vi "VI_unlock.vi"(6 "Verify salt (T)":bool=TRUE, 7 "Remove lib password (T)":bool=TRUE, 8 "error in (no error)":errorcluster, 9 "New Password (\"\")":string, 10 "Output file":path, 11 "Input file":path) -> (0 "error out":errorcluster, 1 "Hash1 salt":string, 2 "Icon":picture, 3 "Version string":string, 4 "Bruteforced salt":bool)   [LabVIEW 2020]
uses:
  <vilib>/Utility/error.llb/Trim Whitespace One-Sided.vi
panel:
  # "(Disable to repair broken BDPW hashes)"
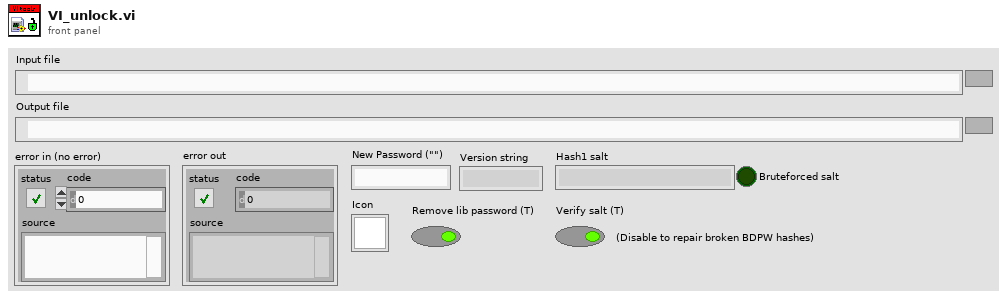
[diagram p1: front panel]
types:
  T1 = cluster{"Major":u8, "Minor":u8, "Fix":u8, "Build":u8}
  T2 = enum16{"open", "replace", "create", "open or create", "replace or create", "replace or create with confirmation"}
  T3 = map{string, cluster{"Offset":i32, "Data":string}}
  T4 = cluster{"Hash1 raw (no salt)":string, "Hash1 (MD5)":string}
  T5 = cluster{"version":u32, "Flags":u32, "viFlags2":u32, "viFlags0C":u32, "viFlags10":u32, "buttonsHidden":u16, "frontpFlags":u16, "instrState":u32, "execState":u32, "execPrio":u16, "viType":u16, "prefExecSyst":i32, "field28":u32, "field2C":u32, "field30":u32, "viSignatureHi":u64, "viSignatureLo":u64, "alignGridFP":u32, "alignGridBD":u32, "field4C":u16, "ctrlIndStyle":u16, "field50_md5Hi":u64, "field50_md5Lo":u64, "libHi":u64, "libLo":u64}
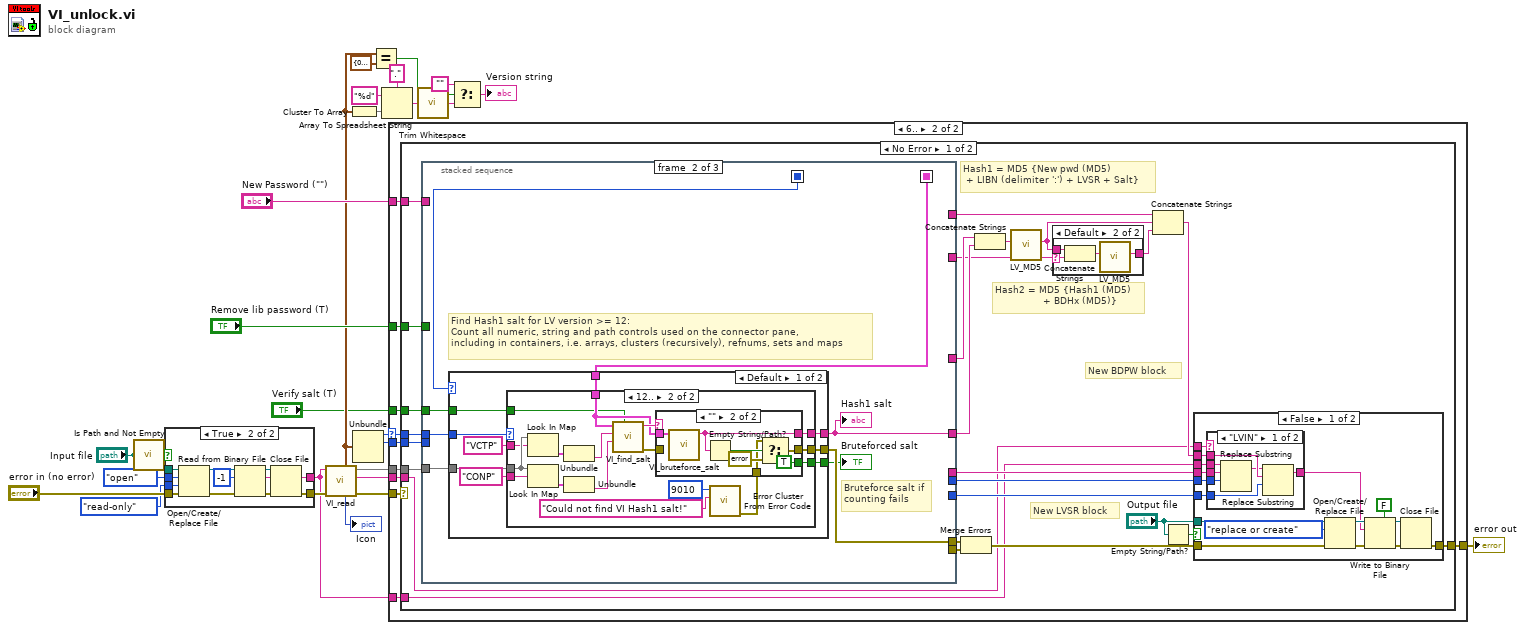
[diagram p0: block diagram]
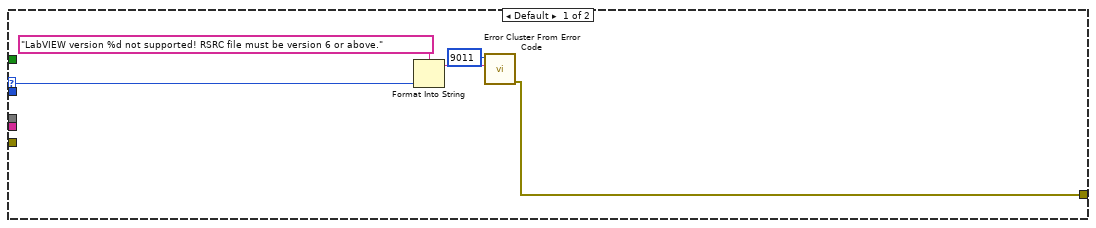
[diagram p2: hidden frame]
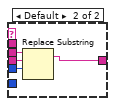
[diagram p4: hidden frame]
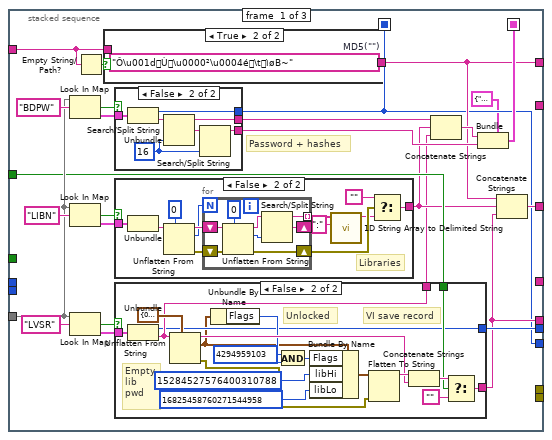
[diagram p6: hidden frame]
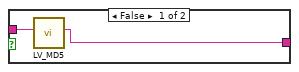
[diagram p7: hidden frame]
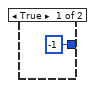
[diagram p8: hidden frame]
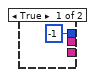
[diagram p10: hidden frame]
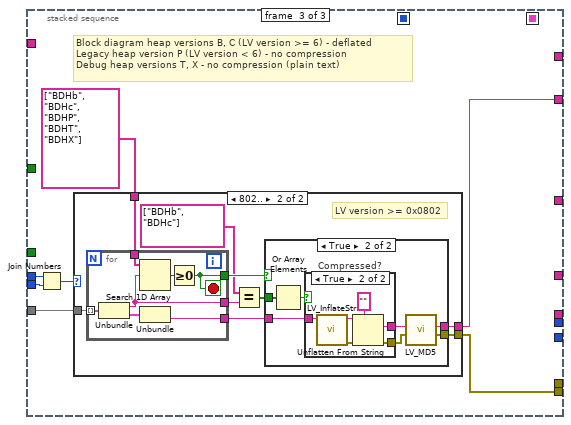
[diagram p14: hidden frame]
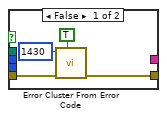
[diagram p19: hidden frame]
diagram:
  n1 = call <vilib>:"Is Path and Not Empty.vi"("path"="Input file") -> ("Is Path and Not Empty?"=w19:bool)  [unwired: 4 in]
  n2 = case "Empty?" shown="True" w19 {
    tunnel: "error in (no error)" -> [w31 w42]
    tunnel: "Input file" -> [_ w41]
    tunnel: [w28 w32] -> w27
    tunnel: enum16{"read/write", "read-only", "write-only"}."read-only" ("access (0:read/write)") -> [_ w40]
    tunnel: T2."open" ("operation (0:open)") -> [_ w39]
    tunnel: [_ w35] -> w5
    frame False {
      n3 = call <vilib>:"Error Cluster From Error Code.vi"("show call chain? (False)"=TRUE, "error in (no error)"=w31, "error code (0)"=1430) -> ("error out"=w28:errorcluster)  [unwired: 6 in]
    }
    frame True {
      n4 = Open/Create/Replace File(file path (use dialog)=w41, error in=w42, operation (0:open)=w39, access (0:read/write)=w40) -> (refnum out=w37:refnum<file>, error out=w38:errorcluster)  [unwired: 2 in, 1 out]
      n5 = Read from Binary File(8:w38, 10:-1 ("count (1)"), 11:w37) -> (0:w33:errorcluster, 2:w35:string, 3:w34:refnum<file>)  [unwired: 3 in, 1 out]
      n6 = Close File(refnum=w34, error in=w33) -> (error out=w32:errorcluster)  [unwired: 1 out]
    }
  }
  n7 = call "VI_read.vi"("error in (no error)"=w27, "File bytestream"=w5) -> ("error out"=w23:errorcluster, "Resource type"=w18:string, "Blocks"=w21:T3, "Icon"=→"Icon":picture, "Version"=w4:T1)  [unwired: 5 in]
  n8 = Cluster To Array(cluster=w4) -> (array=w12:u8[])
  n9 = Unbundle(w4) -> ("Major"=w3:u8, "Minor"=w2:u8)  [unwired: 2 out]
  n10 = Equal?(x=w4, y=T1 {"Major"=0, "Minor"=0, "Fix"=0, "Build"=0}) -> (x = y?=w10:bool)
  n11 = Array To Spreadsheet String(delimiter (Tab)=".", array=w12, 3:"%d" ("format string")) -> (spreadsheet string=w13:string)
  n12 = case shown="6.." w3 {
    selector: w3 -> [w45 w50]
    tunnel: w23 -> [_ w57]
    tunnel: [w43 w56] -> w22
    tunnel: w21 -> [_ w55]
    tunnel: w18 -> [_ w54]
    tunnel: "New Password (\"\")" -> [_ w53]
    tunnel: "Remove lib password (T)" -> [_ w52]
    tunnel: w5 -> [_ w51]
    tunnel: w2 -> [_ w49]
    tunnel: "Verify salt (T)" -> [_ w48]
    frame Default {
      n13 = Format Into String(format string="LabVIEW version %d not supported! RSRC file must be version 6 or above.", w45) -> (resulting string=w44:string)  [unwired: 2 in, 1 out]
      n14 = call <vilib>:"Error Cluster From Error Code.vi"("error message (\"\")"=w44, "error code (0)"=9011) -> ("error out"=w43:errorcluster)  [unwired: 7 in]
    }
    frame 6.. {
      n15 = case shown="No Error" w57 {
        selector: w57 -> [_ w269]
        tunnel: w55 -> [w71 _]
        tunnel: w54 -> [w61 _]
        tunnel: [w62 w269] -> w56
        tunnel: w50 -> [w66 _]
        tunnel: w53 -> [w70 _]
        tunnel: w52 -> [w69 _]
        tunnel: w51 -> [w60 _]
        tunnel: w49 -> [w59 _]
        tunnel: w48 -> [w58 _]
        frame No Error {
          # "New BDPW block"
          # "New LVSR block"
          # "Hash2 = MD5 {Hash1 (MD5)\n                + BDHx (MD5)}"
          # "Hash1 = MD5 {New pwd (MD5)\n + LIBN (delimiter ':') + LVSR + Salt}"
          n16 = stacked-sequence {
            seq-local: [w121 _ _] -> [_ w194 _]
            seq-local: [w116 _ _] -> [_ w190 _]
            tunnel: [_ w192 _] -> w76
            tunnel: w70 -> [w124 _ _]
            tunnel: [_ _ w238] -> w65
            tunnel: [w126 _ _] -> w78
            tunnel: [w119 _ _] -> w77
            tunnel: [w116 _ _] -> w64
            tunnel: [_ _ w237] -> w81
            tunnel: w71 -> [w131 w193 w236]
            tunnel: w69 -> [w127 _ _]
            tunnel: [w118 _ _] -> w68
            tunnel: [w117 _ _] -> w67
            tunnel: w66 -> [_ w196 w234]
            tunnel: [_ w195 _] -> w82
            tunnel: w59 -> [_ _ w233]
            tunnel: w58 -> [_ w189 _]
            frame #0 {
              # "Password + hashes"
              n17 = Look In Map(map=w131, key="BDPW") -> (key not found?=w137:bool, value=w136:cluster{"Offset":i32, "Data":string})  [unwired: 1 in]
              n18 = Look In Map(map=w131, key="LIBN") -> (key not found?=w134:bool, value=w133:cluster{"Offset":i32, "Data":string})  [unwired: 1 in]
              n19 = Look In Map(map=w131, key="LVSR") -> (key not found?=w129:bool, value=w128:cluster{"Offset":i32, "Data":string})  [unwired: 1 in]
              n20 = Empty String/Path?(string/path=w124) -> (empty?=w125:bool)
              n21 = case shown="True" w125 {
                tunnel: w124 -> [w140 _]
                tunnel: [w139 w141] -> w118
                frame False {
                  n22 = call "LV_MD5.vi"("Input string"=w140) -> ("MD5 digest (16-bytes)"=w139:string)  [unwired: 9 in, 1 out]
                }
                frame True {
                  w141 = "Ô\u001dÙ\u0000²\u0004é\tìøB~"  # MD5("")
                }
              }
              n23 = case "Has BDPW?" shown="False" w137 {
                tunnel: w136 -> [_ w188]
                tunnel: [-1 ("Offset") w187] -> w116
                tunnel: [_ w183] -> w130
                tunnel: [_ w182] -> w122
                frame True {
                }
                frame False {
                  w184 = 16 ("offset (0)")
                  n24 = Unbundle(w188) -> ("Offset"=w187:i32, "Data"=w186:string)
                  n25 = Search/Split String(string=w186, offset (0)=w184) -> (substring before match=w183:string, match + rest of string=w185:string)  [unwired: 1 in, 1 out]
                  n26 = Search/Split String(string=w185, offset (0)=w184) -> (substring before match=w182:string)  [unwired: 1 in, 2 out]
                }
              }
              n27 = case "Has LIBN?" shown="False" w134 {
                tunnel: w133 -> [_ w168]
                tunnel: [_ w161] -> w120
                frame True {
                }
                frame False {
                  # "Libraries"
                  n28 = Unbundle(w168) -> ("Data"=w167:string)  [unwired: 1 out]
                  n29 = Unflatten From String(type=0 ("I32"), binary string=w167) -> (rest of the binary string=w170:string, value=w169:i32, error out=w171:errorcluster)  [unwired: 3 in]
                  n30 = for {
                    N: w169 -> [_]
                    shift-right: [w174] -> _
                    shift-left: w170 -> [w178]
                    shift-right: [w175] -> w164
                    shift-left: w171 -> [w179]
                    tunnel: [w173] -> w166 mode=indexing
                    n31 = Unflatten From String(type=u8 0 ("U8"), binary string=w178, error in (no error)=w179) -> (rest of the binary string=w177:string, value=w176:u8, error out=w175:errorcluster)  [unwired: 2 in]
                    n32 = Search/Split String(string=w177, offset (0)=w176) -> (substring before match=w173:string, match + rest of string=w174:string)  [unwired: 1 in, 1 out]
                  }
                  n33 = call <vilib>:"1D String Array to Delimited String.vi"("delimiter"=":", "string array"=w166) -> ("delimited string"=w163:string)  [unwired: 9 in]
                  n34 = Select(t="", s=w164, f=w163) -> (s? t:f=w161:string)
                }
              }
              n35 = case "Has LIBN?" shown="False" w129 {
                tunnel: w128 -> [_ w150]
                tunnel: [_ w146] -> w117
                tunnel: w127 -> [_ w148]
                tunnel: [-1 ("Offset") w144] -> w126
                tunnel: [_ w149] -> w115
                frame True {
                }
                frame False {
                  # "VI save record"
                  # "Unlocked"
                  # "Empty\nlib\npwd"
                  n36 = Unbundle(w150) -> ("Offset"=w144:i32, "Data"=w149:string)
                  n37 = Unflatten From String(type=T5 {"version"=0, "Flags"=0, "viFlags2"=0, "viFlags0C"=0, "viFlags10"=0, "buttonsHidden"=0, "frontpFlags"=0, "instrState"=0, "execState"=0, "execPrio"=0, "viType"=0, "prefExecSyst"=0, "field28"=0, "field2C"=0, "field30"=0, "viSignatureHi"=0, "viSignatureLo"=0, "alignGridFP"=0, "alignGridBD"=0, "field4C"=0, "ctrlIndStyle"=0, "field50_md5Hi"=0, "field50_md5Lo"=0, "libHi"=0, "libLo"=0} ("LVSR"), binary string=w149) -> (rest of the binary string=w157:string, value=w143:T5, error out=w145:errorcluster)  [unwired: 3 in]
                  n38 = Unbundle By Name(w143) -> ("Flags"=w147:u32)
                  n39 = And(x=u32 4294959103 ("Unlocked"), y=w147) -> (x .and. y?=w151:u32)
                  n40 = Bundle By Name(cluster=w143, "Flags"=w151, "libHi"=u64 15284527576400310788 ("libpass_md5Hi"), "libLo"=u64 16825458760271544958 ("libpass_md5Lo")) -> (w156:T5)
                  n41 = Flatten To String(anything=w156, error in (no error)=w145) -> (data string=w158:string)  [unwired: 2 in, 2 out]
                  n42 = Concatenate Strings(w158, w157) -> (w160:string)
                  n43 = Select(t=w160, s=w148, f="") -> (s? t:f=w146:string)
                }
              }
              n44 = Concatenate Strings(w130, w120, w115) -> (w123:string)
              n45 = Bundle(cluster=T4 {"Hash1 raw (no salt)"="", "Hash1 (MD5)"=""} ("output cluster"), "Hash1 raw (no salt)"=w123, "Hash1 (MD5)"=w122) -> (w121:T4)
              n46 = Concatenate Strings(w118, w120, w117) -> (w119:string)
            }
            frame #1 {
              # "Bruteforce salt if\ncounting fails"
              # "Find Hash1 salt for LV version >= 12:\nCount all numeric, string and path controls used on the connector pane,\nincluding in containers, i.e. arrays, clusters (recursively), refnums, sets and maps"
              n47 = case shown="Default" w190 {
                tunnel: [w205 _] -> w192
                tunnel: w196 -> [w202 _]
                tunnel: [w204 _] -> w195
                tunnel: w194 -> [w203 _]
                tunnel: w193 -> [w201 _]
                tunnel: [w199 _] -> w191
                tunnel: w189 -> [w197 _]
                frame Default {
                  n48 = case shown="12.." w202 {
                    tunnel: [_ w217] -> w205
                    tunnel: w203 -> [_ w207]
                    tunnel: [_ w218] -> w204
                    tunnel: w201 -> [_ w212]
                    tunnel: "CONP" ("key") -> [_ w221]
                    tunnel: [_ w213] -> w199
                    tunnel: "VCTP" ("key") -> [_ w211]
                    tunnel: w197 -> [_ w206]
                    frame Default {
                    }
                    frame 12.. {
                      n49 = Look In Map(map=w212, key=w211) -> (value=w210:cluster{"Offset":i32, "Data":string})  [unwired: 1 in, 1 out]
                      n50 = Look In Map(map=w212, key=w221) -> (value=w222:cluster{"Offset":i32, "Data":string})  [unwired: 1 in, 1 out]
                      n51 = Unbundle(w210) -> ("Data"=w209:string)  [unwired: 1 out]
                      n52 = Unbundle(w222) -> ("Data"=w208:string)  [unwired: 1 out]
                      n53 = call "VI_find_salt.vi"("Verify salt (T)"=w206, "CONP block"=w208, "VCTP block"=w209, "Hashes"=w207) -> ("error out"=w219:errorcluster, "Salt"=w220:string)  [unwired: 6 in]
                      n54 = call <vilib>:"Error Cluster From Error Code.vi"("error message (\"\")"="Could not find VI Hash1 salt!" ("error message (\"\")"), "error code (0)"=9010) -> ("error out"=w214:errorcluster)  [unwired: 7 in]
                      n55 = case shown="\"\"" w220 {
                        selector: w220 -> [w223 _]
                        tunnel: [w224 w226] -> w218
                        tunnel: w219 -> [w224 _]
                        tunnel: [w223 w230] -> w217
                        tunnel: w207 -> [_ w231]
                        tunnel: w214 -> [_ w227]
                        tunnel: [_ TRUE] -> w213
                        frame Default {
                        }
                        frame "" {
                          n56 = call "VI_bruteforce_salt.vi"("Hashes"=w231) -> ("Salt"=w230:string)  [unwired: 10 in]
                          n57 = Empty String/Path?(string/path=w230) -> (empty?=w229:bool)
                          n58 = Select(t=w227, s=w229, f=errorcluster {"status"=FALSE, "code"=0, "source"=""}) -> (s? t:f=w226:errorcluster)
                        }
                      }
                    }
                  }
                }
                frame ..-1 {
                  # "No BDPW block (global variables, controls etc.)"
                }
              }
              "Hash1 salt" <- w192
              "Bruteforced salt" <- w191
            }
            frame #2 {
              # "Block diagram heap versions B, C (LV version >= 6) - deflated\nLegacy heap version P (LV version < 6) - no compression\nDebug heap versions T, X - no compression (plain text)"
              n59 = Join Numbers(hi=w234, lo=w233) -> ((hi.lo)=w235:u16)
              n60 = case shown="802.." w235 {
                tunnel: [_ w246] -> w238
                tunnel: [_ w245] -> w237
                tunnel: w236 -> [_ w244]
                tunnel: string[] ["BDHb", "BDHc", "BDHP", "BDHT", "BDHX"] -> [_ w239]
                frame Default {
                  # "LV version < 8.2: No Hash2"
                }
                frame 2050.. {
                  # "LV version >= 0x0802"
                  n61 = for {
                    tunnel: w244 -> [w252] mode=indexing
                    tunnel: [w251] -> w243
                    tunnel: [w249] -> w242
                    tunnel: [w253] -> w241
                    tunnel: w239 -> [w248]
                    stop <- w249 stop-if-true
                    n62 = Unbundle(w252) -> (w251:string, "value"=w254:cluster{"Offset":i32, "Data":string})
                    n63 = Search 1D Array(1D array=w248, element=w251) -> (index of element=w250:i32)  [unwired: 1 in]
                    n64 = Unbundle(w254) -> ("Data"=w253:string)  [unwired: 1 out]
                    n65 = Greater Or Equal To 0?(x=w250) -> (x >= 0?=w249:bool)
                  }
                  n66 = Equal?(x=string[] ["BDHb", "BDHc"], y=w243) -> (x = y?=w247:bool[])
                  n67 = case shown="True" w242 {
                    tunnel: w247 -> [_ w261]
                    tunnel: w241 -> [_ w259]
                    tunnel: [_ w256] -> w245
                    tunnel: [_ w255] -> w246
                    frame False {
                    }
                    frame True {
                      n68 = Or Array Elements(Boolean array=w261) -> (logical OR=w260:bool)
                      n69 = case "Compressed?" shown="True" w260 {
                        tunnel: w259 -> [w262 w266]
                        tunnel: [_ w268] -> w257
                        tunnel: [w262 w267] -> w258
                        frame False {
                        }
                        frame True {
                          n70 = call "LV_InflateStr.vi"("Deflated string with size header"=w266) -> ("error out"=w264:errorcluster, "Inflated string"=w265:string)  [unwired: 9 in]
                          n71 = Unflatten From String(type="", binary string=w265, error in (no error)=w264) -> (value=w267:string, error out=w268:errorcluster)  [unwired: 2 in, 1 out]
                        }
                      }
                      n72 = call "LV_MD5.vi"("error in (no error)"=w257, "Input string"=w258) -> ("error out"=w256:errorcluster, "MD5 digest (16-bytes)"=w255:string)  [unwired: 8 in]
                    }
                  }
                }
              }
            }
          }
          n73 = Merge Errors(w82, w81) -> (w63:errorcluster)
          n74 = Concatenate Strings(w77, w76) -> (w74:string)
          n75 = call "LV_MD5.vi"("Input string"=w74) -> ("MD5 digest (16-bytes)"=w73:string)  [unwired: 9 in, 1 out]
          n76 = case shown="Default" w65 {
            selector: w65 -> [_ w83]
            tunnel: w73 -> [_ w86]
            tunnel: [_ w84] -> w72
            frame "" {
            }
            frame Default {
              n77 = Concatenate Strings(w86, w83) -> (w85:string)
              n78 = call "LV_MD5.vi"("Input string"=w85) -> ("MD5 digest (16-bytes)"=w84:string)  [unwired: 9 in, 1 out]
            }
          }
          n79 = Concatenate Strings(w68, w73, w72) -> (w75:string)
          n80 = Empty String/Path?(string/path="Output file") -> (empty?=w80:bool)
          n81 = case shown="False" w80 {
            tunnel: [w95 _] -> w62
            tunnel: "Output file" -> [w94 _]
            tunnel: w60 -> [w93 _]
            tunnel: w61 -> [w92 _]
            tunnel: w64 -> [w87 _]
            tunnel: w75 -> [w91 _]
            tunnel: w78 -> [w90 _]
            tunnel: w67 -> [w89 _]
            tunnel: w63 -> [w88 _]
            frame False {
              n82 = case shown="\"LVIN\"" w92 {
                tunnel: w93 -> [w105 w113]
                tunnel: [w103 w110] -> w96
                tunnel: w91 -> [w109 _]
                tunnel: w90 -> [w107 w111]
                tunnel: w89 -> [w108 w112]
                tunnel: w87 -> [w106 _]
                frame "LVIN" {
                  n83 = Replace Substring(3:w107, 4:w108, 5:w105) -> (1:w104:string)  [unwired: 1 in, 1 out]
                  n84 = Replace Substring(3:w106, 4:w109, 5:w104) -> (1:w103:string)  [unwired: 1 in, 1 out]
                }
                frame Default {
                  n85 = Replace Substring(3:w111, 4:w112, 5:w113) -> (1:w110:string)  [unwired: 1 in, 1 out]
                }
              }
              n86 = Open/Create/Replace File(file path (use dialog)=w94, error in=w88, operation (0:open)=T2."replace or create") -> (refnum out=w98:refnum<file>, error out=w101:errorcluster)  [unwired: 1 in, 3 out]
              n87 = Write to Binary File(file (use dialog)=w98, data=w96, error in=w101, 5:FALSE ("prepend array or string size? (T)")) -> (refnum out=w100:refnum<file>, error out=w99:errorcluster)  [unwired: 2 in, 1 out]
              n88 = Close File(refnum=w100, error in=w99) -> (error out=w95:errorcluster)  [unwired: 1 out]
            }
            frame True {
            }
          }
        }
        frame Default {
        }
      }
    }
  }
  "error out" <- w22
  n89 = call <vilib>:"Trim Whitespace.vi"("string"=w13) -> ("trimmed string"=w9:string)  [unwired: 1 in]
  n90 = Select(t="", s=w10, f=w9) -> (s? t:f=→"Version string":string)
